vi "MWG.vi"(0 "System no.":i32=1 min=1 max=4 step=1, 2 "Axes to move":string[](array[string]), 3 "Position values":dbl[](array[numeric]) format="%.6f", 4 "No.of digits":i16=4, 5 "error in":errorcluster) -> (19 "error out":errorcluster)   [LabVIEW 2020]
doc: "Moves specified axes to absolute position without updating graphics on the controller screen (fast move). No. of digits is the number of digits after the decimal point in the position value(s) that will be sent. Required by 1D Scan.vi and 2D Scan.vi.\n\nF-206: Only for GCS syntax version = GCS 1.0 (Check with CSV?.vi. If CSV?.vi is not supported, syntax version is GCS 1.0). No mix between F-206 axes X,Y,Z,U,V,W ,separate axes A,B and NanoCube axes K,L,M allowed. For compatibility reasons, VI calls MOV.vi if GCS syntax version is > GCS 1.0.\n\nC-887, M-8X0: Only for GCS syntax version = GCS 1.0 (Check with CSV?.vi. If CSV?.vi is not supported, syntax version is GCS 1.0) and only for controllers based on C-842.80. If not supported, must be present anyway. For compatibility reasons, VI calls MOV.vi if GCS syntax version is > GCS 1.0."
uses:
  Syntax.ctl
  Global1.vi
panel:
  # "Moves stage to absolute position without updating graphics\non the controller screen (fast move)."
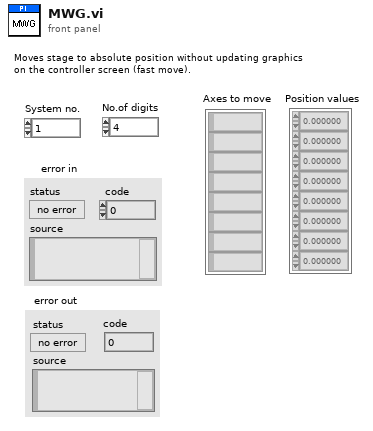
[diagram p1: front panel]
types:
  T1 = typedef "Syntax.ctl" = enum16{"GCS 1.0", "GCS 2.0", "GCS 3.0"}
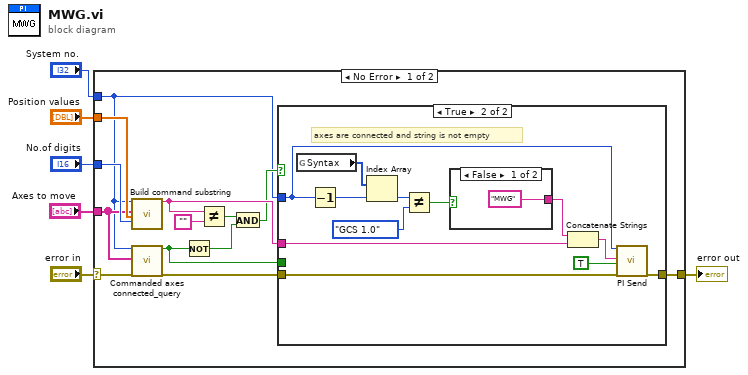
[diagram p0: block diagram]
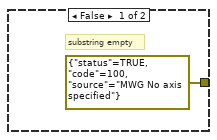
[diagram p3: hidden frame]
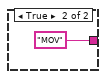
[diagram p4: hidden frame]
diagram:
  n1 = case shown="No Error" "error in" {
    selector: "error in" -> [w7 w39]
    tunnel: [w19 w39] -> w6
    tunnel: "Position values" -> [w16 _]
    tunnel: "No.of digits" -> [w15 _]
    tunnel: "System no." -> [w8 _]
    tunnel: "Axes to move" -> [w13 _]
    frame No Error {
      n2 = call "Build command substring.vi"("System no."=w8, "Affected axes"=w13, "Parameters"=w16, "No. of digits"=w15) -> ("Command substring"=w17:string)  [unwired: 3 in, 12 out]
      n3 = call "Commanded axes connected_query.vi"("System no."=w8, "Commanded axes"=w13, "error in"=w7) -> ("Controller error"=w11:bool, "error out"=w14:errorcluster)  [unwired: 1 in, 14 out]
      n4 = Not(x=w11) -> (.not. x?=w10:bool)
      n5 = Not Equal?(x=w17, y="") -> (x != y?=w12:bool)
      n6 = And(x=w12, y=w10) -> (x .and. y?=w9:bool)
      n7 = case shown="True" w9 {
        tunnel: w17 -> [_ w35]
        tunnel: [w22 w31] -> w19
        tunnel: w14 -> [w20 w32]
        tunnel: w11 -> [w21 _]
        tunnel: w8 -> [_ w26]
        frame False {
          # "substring empty or axis not connected"
          n8 = case shown="True" w21 {
            tunnel: [errorcluster {"status"=TRUE, "code"=100, "source"="MWG No axis specified"} ("error out") w24] -> w22
            tunnel: w20 -> [_ w24]
            frame False {
              # "substring empty"
            }
            frame True {
              # "commanded axis not connected"
            }
          }
        }
        frame True {
          # "axes are connected and string is not empty"
          n9 = global read "Global1.vi" "Syntax"() -> (w30:T1[])
          n10 = Decrement(x=w26) -> (x-1=w29:i32)
          n11 = Index Array(array=w30, index=w29) -> (element=w28:T1)
          n12 = Not Equal?(x=w28, y=Syntax."GCS 1.0") -> (x != y?=w27:bool)
          n13 = case shown="False" w27 {
            tunnel: ["MWG" "MOV"] -> w36
            frame False {
            }
            frame True {
            }
          }
          n14 = Concatenate Strings(w36, w35) -> (w33:string)
          n15 = call "PI Send.vi"("System no."=w26, "String to send"=w33, "Attach termination char.?"=TRUE ("Attach Linefeed?"), "error in"=w32) -> ("error out"=w31:errorcluster)  [unwired: 2 in, 13 out]
        }
      }
    }
    frame Error {
    }
  }
  "error out" <- w6
